vi "New Button Test.vi"() -> ()   [LabVIEW 2016]
panel:
  in  "Stop Button":bool
  out "Boolean array":bool[](array[boolean])
  in  "String":string
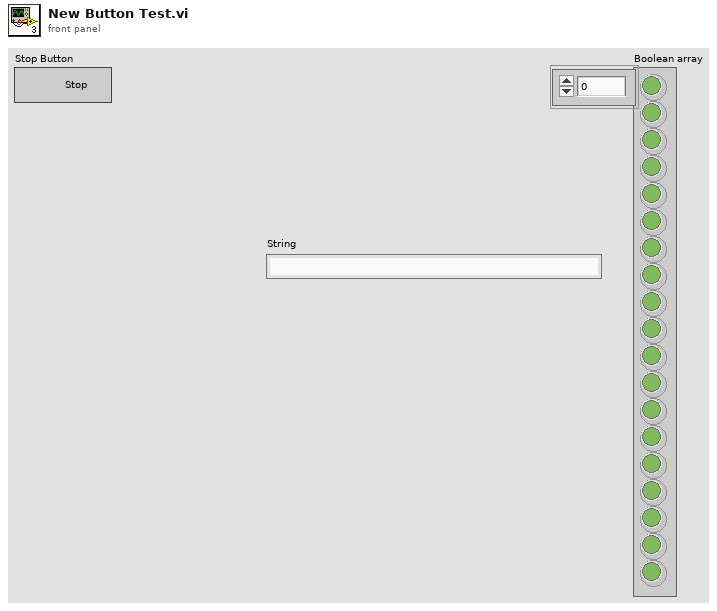
[diagram p1: front panel]
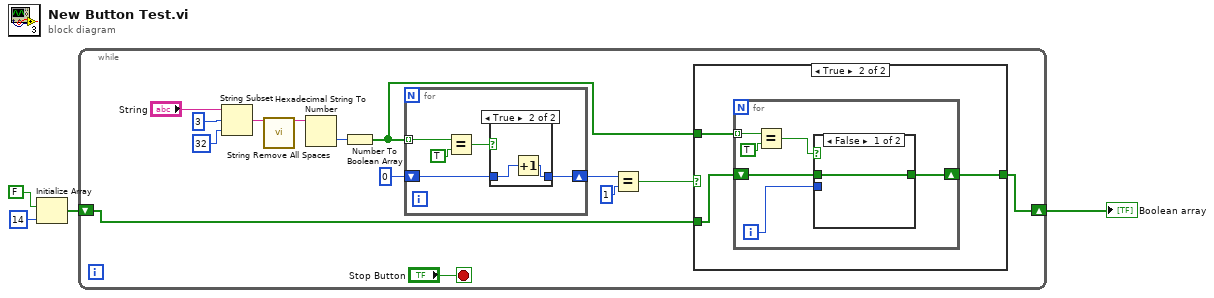
[diagram p0: block diagram]
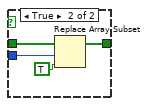
[diagram p3: hidden frame]
diagram:
  n1 = Initialize Array(FALSE, 14 ("dimension size")) -> (w1:bool[])
  n2 = while {
    shift-right: [w6] -> w4
    shift-left: w1 -> [w5]
    stop <- "Stop Button" stop-if-true
    n3 = String Subset(string="String", offset (0)=3, length (rest)=32 ("length (rest)")) -> (substring=w15:string)
    n4 = call "String Remove All Spaces.vi"("Input String"=w15) -> ("Spaces Removed"=w14:string)  [unwired: 13 in, 1 out]
    n5 = Hexadecimal String To Number(string=w14) -> (number=w13:u32)  [unwired: 2 in, 1 out]
    n6 = Number To Boolean Array(number=w13) -> (Boolean array=w7:bool[])
    n7 = for {
      tunnel: w7 -> [w34] mode=indexing
      shift-right: [w37] -> w10
      shift-left: 0 -> [w38]
      n8 = Equal?(x=w34, y=TRUE) -> (x = y?=w35:bool)
      n9 = case shown="True" w35 {
        tunnel: w38 -> [w39 w41]
        tunnel: [w39 w40] -> w37
        frame False {
        }
        frame True {
          n10 = Increment(x=w41) -> (x+1=w40:i32)
        }
      }
    }
    n11 = Equal?(x=w10, y=1) -> (x = y?=w8:bool)
    n12 = case shown="True" w8 {
      tunnel: w7 -> [_ w22]
      tunnel: [w19 w21] -> w6
      tunnel: w5 -> [w19 w20]
      frame False {
      }
      frame True {
        n13 = for {
          tunnel: w22 -> [w27] mode=indexing
          shift-right: [w25] -> w21
          shift-left: w20 -> [w24]
          i -> [w26]
          n14 = Equal?(x=w27, y=TRUE) -> (x = y?=w23:bool)
          n15 = case shown="False" w23 {
            tunnel: w26 -> [_ w33]
            tunnel: [w29 w31] -> w25
            tunnel: w24 -> [w29 w30]
            frame False {
            }
            frame True {
              n16 = Replace Array Subset(array=w30, new element=TRUE ("new element/subarray"), index=w33) -> (w31:bool[])
            }
          }
        }
      }
    }
  }
  "Boolean array" <- w4
